vi "適應性控制(實際控制).vi"() -> ()   [LabVIEW 2010]
panel:
  in  "number of samples(不可低於2)":i32=100 min=2
  out "while 每次運行時間(ms)":u32
  in  "rate":dbl=1000.0
  out "收斂時間(s)":dbl
  out "收斂燈":bool
  in  "ERR誤差低於多少V亮燈":dbl=0.05
  out "ERR message":string=" INSTRUCTIONS:\r\rNormal Use:  When using subVIs that incorporate the error in/error out (or error I/O) structure, place this handler where you want to inform the user of an error, typically at the end of the I/O data path, as the last action of the program.  If the error in error? is ERROR, the handler creates a message describing the error and its source.  If the type of dialog = 1 (default), the message is displayed to the user, who can only acknowedge it.  If the type = 2, the user can acknowledge the message or abort execution; aborting a program with active I/O is not recommended.  If the type = 0, no message is displayed; this is used to process the error programmatically, and the error out cluster elements are wired to individual terminals for that reason.  \r\rOther Use:\n\r\nlocal testing.  To test the error code of a subVI or function that does not have the error I/O structure, you can wire its error code and a source string to the local error code and error source inputs.  If error in error? indicates no error and error code is not equal to 0, the local code and source are substituted for the error in values, and error? is set TRUE (ERROR)."
  out "理想系統與FIR輸出":cluster{dbl, dbl}(graph)
  out "system輸出":dbl
  out "input_x(t)":dbl(graph)
  out "ERR":dbl(graph)
  out "權重函數向量":dbl[](array[numeric])
  in  "order":i32=8
  out "LMS":dbl[](graph)
  out "FIR輸出":dbl
  in  "Stop Button":bool
  in  "u(收斂係數)":dbl=0.005
  # "A0:模擬輸入 pulse_output 1"
  # "A1:理想系統 pulse_output 2"
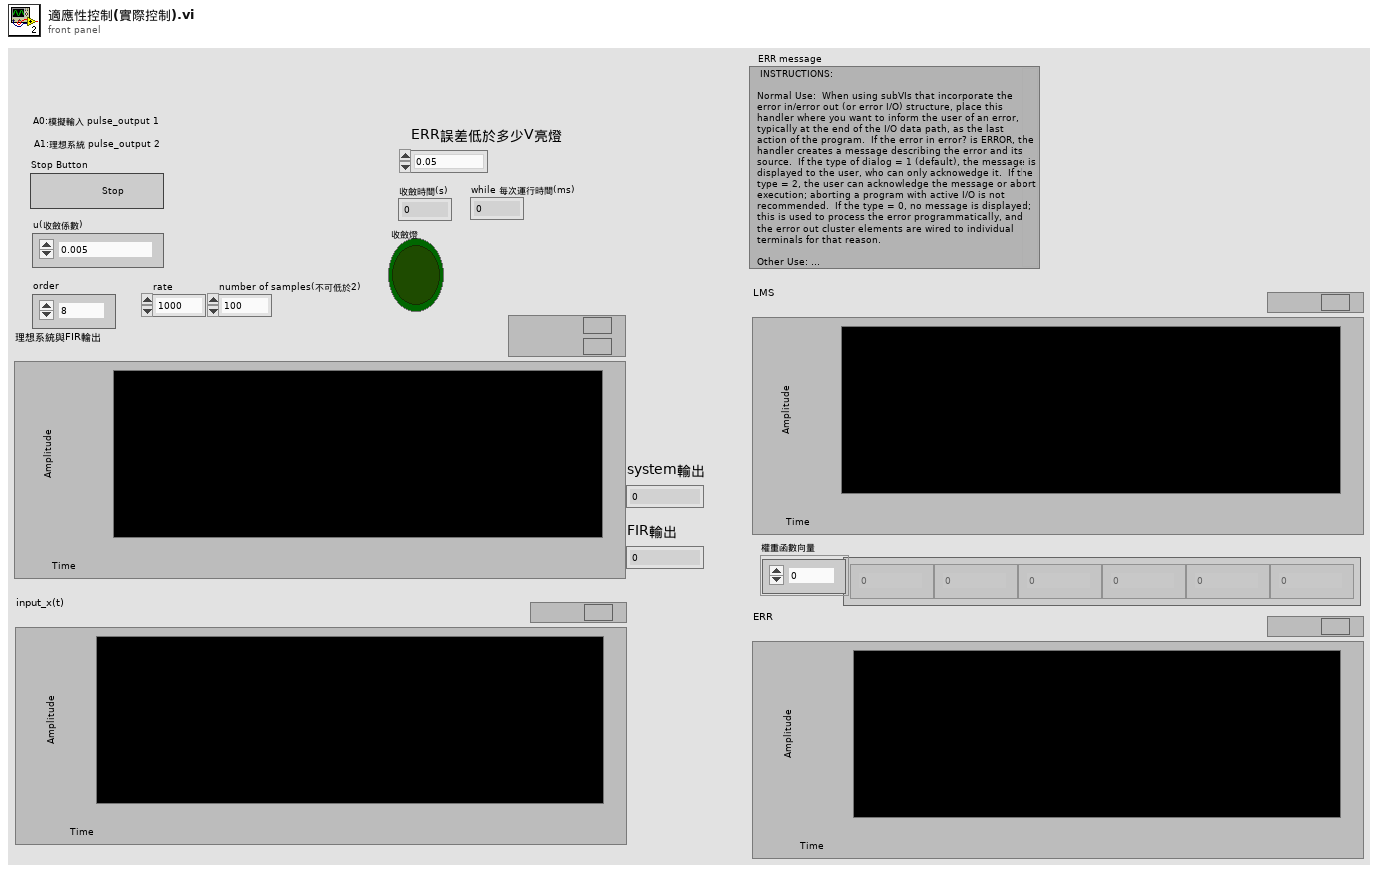
[diagram p1: front panel]
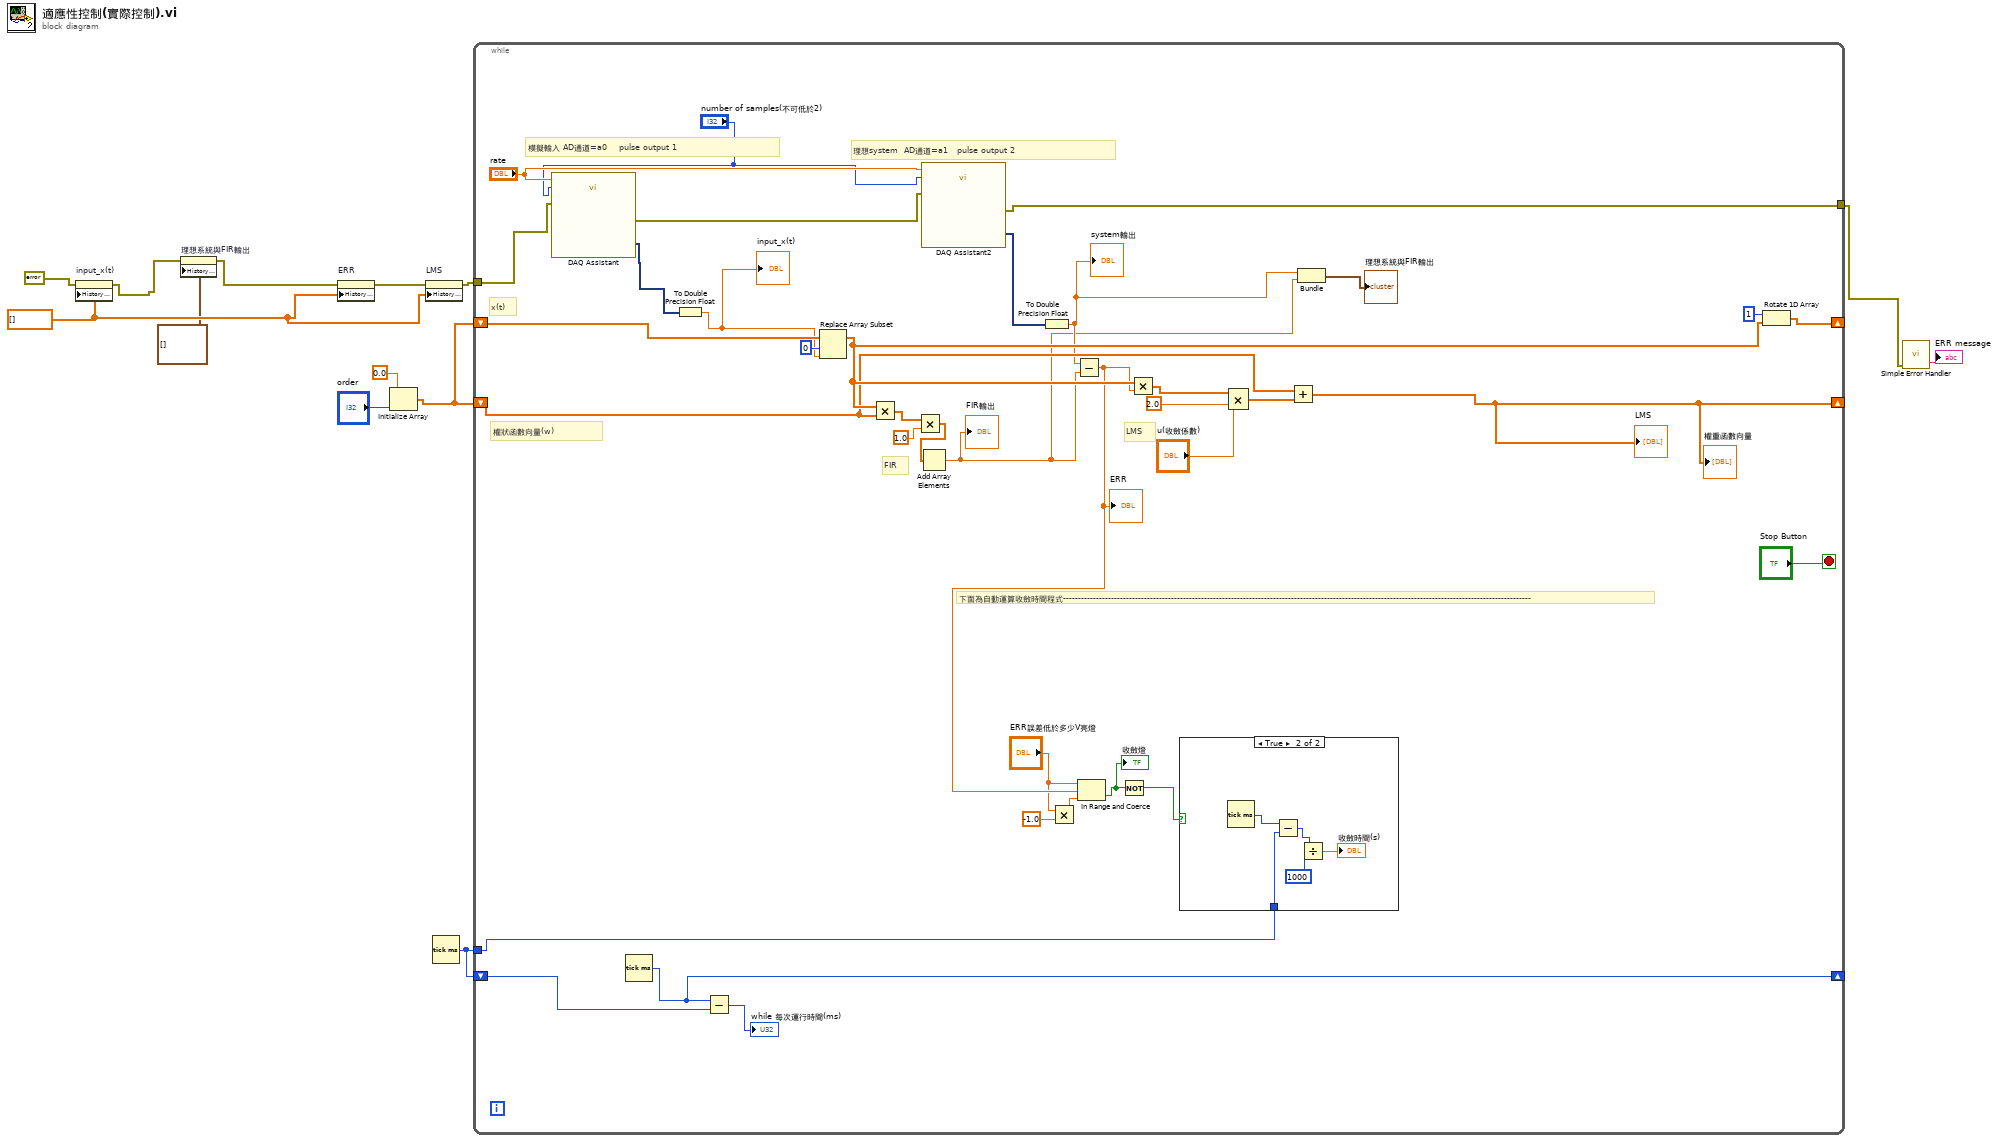
[diagram p0: block diagram]
diagram:
  w9 = dbl[] [] ("History Data")
  n1 = property on="input_x(t)" class="WFChart (strict)"(error in=errorcluster {"status"=FALSE, "code"=0, "source"=""} ("error constant"), "History Data"=w9) -> (error out=w6:errorcluster)  [unwired: 1 in, 1 out]
  n2 = property on="理想系統與FIR輸出" class="WFChart (strict)"(error in=w6, "History Data"=cluster{dbl, dbl}[] []) -> (error out=w5:errorcluster)  [unwired: 1 in, 1 out]
  n3 = property on="ERR" class="WFChart (strict)"(error in=w5, "History Data"=w9) -> (error out=w7:errorcluster)  [unwired: 1 in, 1 out]
  n4 = Initialize Array "Initialize Array"(0.0 ("element"), "order") -> (w11:dbl[])
  n5 = property on="LMS" class="WFChart (strict)"(error in=w7, "History Data"=w9) -> (error out=w8:errorcluster)  [unwired: 1 in, 1 out]
  n6 = Tick Count (ms)() -> (millisecond timer value=w1:u32)
  n7 = while {
    shift-right: [w40] -> _
    shift-left: w11 -> [w39]
    shift-right: [w36] -> _
    shift-left: w11 -> [w35]
    tunnel: w8 -> [w32]
    tunnel: [w27] -> w3
    shift-right: [w16] -> _
    shift-left: w1 -> [w18]
    tunnel: w1 -> [w17]
    stop <- "Stop Button" stop-if-true
    # "下面為自動運算收斂時間程式------------------------------------------------------------------------------------------------------------------------------------------------------------"
    # "LMS"
    # "FIR"
    # "模擬輸入 AD通道=a0    pulse output 1"
    # "權狀函數向量(w)"
    # "x(t)"
    # "理想system  AD通道=a1   pulse output 2"
    n8 = call "DAQ Assistant"("rate"="rate", "number of samples"="number of samples(不可低於2)", "error in"=w32) -> ("data"=w33:dynamicdata, "error out"=w28:errorcluster)  [unwired: 14 in, 1 out]
    n9 = Tick Count (ms)() -> (millisecond timer value=w16:u32)
    n10 = To Double Precision Float(number=w33) -> (double precision float=w34:dbl)
    "input_x(t)" <- w34
    n11 = Subtract(x=w16, y=w18) -> (x-y=→"while 每次運行時間(ms)":u32)
    n12 = Replace Array Subset "Replace Array Subset"(array=w39, new element=w34, index=0) -> (w37:dbl[])
    n13 = Multiply(x=w37, y=w35) -> (x*y=w49:dbl[])
    n14 = Multiply(x=w49, y=1.0) -> (x*y=w42:dbl[])
    n15 = Add Array Elements(numeric array=w42) -> (sum=w30:dbl)
    "FIR輸出" <- w30
    n16 = call "DAQ Assistant2"("rate"="rate", "number of samples"="number of samples(不可低於2)", "error in"=w28) -> ("data"=w26:dynamicdata, "error out"=w27:errorcluster)  [unwired: 14 in, 1 out]
    n17 = To Double Precision Float(number=w26) -> (double precision float=w31:dbl)
    "system輸出" <- w31
    n18 = Multiply(x="ERR誤差低於多少V亮燈", y=-1.0) -> (x*y=w24:dbl)
    n19 = Subtract(x=w31, y=w30) -> (x-y=w25:dbl)
    "ERR" <- w25
    n20 = In Range and Coerce(upper limit="ERR誤差低於多少V亮燈", x=w25, lower limit=w24) -> (In Range?=w20:bool)  [unwired: 1 out]
    "收斂燈" <- w20
    n21 = Not(x=w20) -> (.not. x?=w21:bool)
    n22 = Multiply(x=w37, y=w25) -> (x*y=w47:dbl[])
    n23 = case shown="True" w21 {
      tunnel: w17 -> [_ w53]
      frame False {
      }
      frame True {
        n24 = Tick Count (ms)() -> (millisecond timer value=w54:u32)
        n25 = Subtract(x=w54, y=w53) -> (x-y=w52:u32)
        n26 = Divide(x=w52, y=u32 1000) -> (x/y=→"收斂時間(s)":dbl)
      }
    }
    n27 = Compound Arithmetic op=MULTIPLY(w47, 2.0 ("value"), "u(收斂係數)") -> (w44:dbl[])
    n28 = Add(x=w35, y=w44) -> (x+y=w36:dbl[])
    "LMS" <- w36
    "權重函數向量" <- w36
    n29 = Bundle(w31, w30) -> (→"理想系統與FIR輸出":cluster{dbl, dbl})  [unwired: 1 in]
    n30 = Rotate 1D Array(1:w37, 2:1 ("n")) -> (0:w40:dbl[])
  }
  n31 = call <vilib>:"Simple Error Handler.vi"("error in (no error)"=w3) -> ("message"=→"ERR message":string)  [unwired: 4 in, 4 out]
